vi "calcMinVel.vi"(1 "velocity2":dbl, 2 "velocity1":dbl) -> (0 "minVal":dbl)   [LabVIEW 2015]
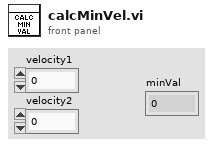
[diagram p1: front panel]
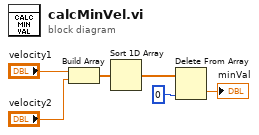
[diagram p0: block diagram]
diagram:
  n1 = Build Array("velocity1", "velocity2") -> (w2:dbl[])
  n2 = Sort 1D Array(array=w2) -> (sorted array=w4:dbl[])
  n3 = Delete From Array(array=w4, index=0) -> (deleted portion=→"minVal":dbl)  [unwired: 1 in, 1 out]
